vi "Set Event HMI.vi"(8 "error in (no error)":errorcluster caption="entrée d'erreur (pas d'erreur)", 10 "Event HMI":T1, 11 "Sequencer (Default) en entrée":refnum<class "Sequencer (Default).lvclass">) -> (0 "error out":errorcluster caption="sortie d'erreur", 3 "Sequencer (Default) en sortie":refnum<class "Sequencer (Default).lvclass">)   [LabVIEW 2020, in "Library Core.lvlib" / "Sequencer (Default).lvclass"]
uses:
  Sequencer (Default).lvclass
  Software/Standard TB/Function/Type DEF/Commande Gestion Execution Scenario.ctl
  Commun VI/TypeDef/Commande Test/Commande Value Type.ctl
  Commun VI/TypeDef/Commande Test/Commande Type Test.ctl
  Sequencer (Default).lvclass/Sequencer (Default).ctl
  Commun VI/Library Commun.lvlib
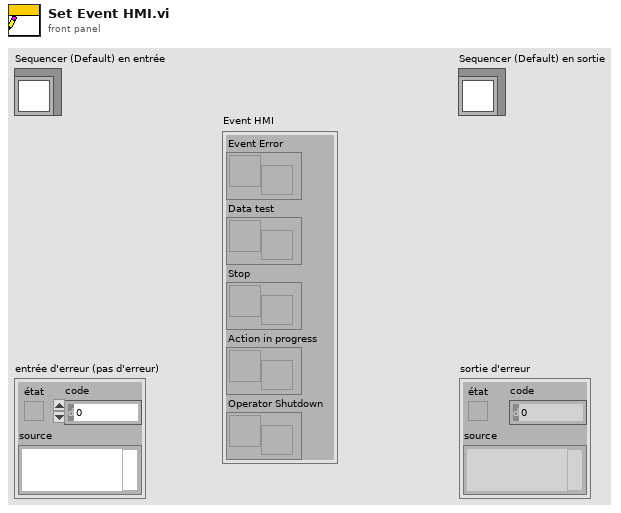
[diagram p1: front panel]
types:
  T1 = cluster{"Event Error":refnum<user-event>, "Data test ":refnum<user-event>, "Stop":refnum<user-event>, "Action in progress":refnum<user-event>, "Operator Shutdown":refnum<user-event>}
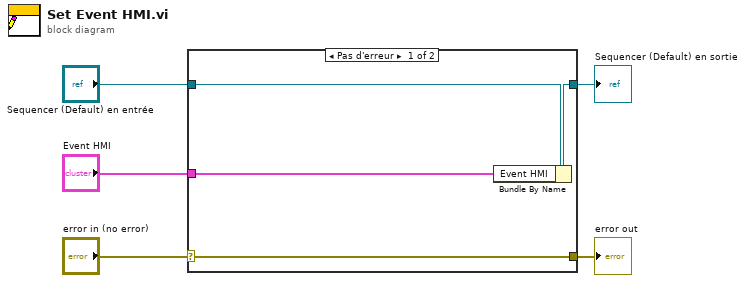
[diagram p0: block diagram]
diagram:
  n1 = case shown="Pas d'erreur" "error in (no error)" {
    selector: "error in (no error)" -> [w9 w10]
    tunnel: [w9 w10] -> w4
    tunnel: [w7 w11] -> w2
    tunnel: "Sequencer (Default) en entrée" -> [w8 w11]
    tunnel: "Event HMI" -> [w6 _]
    frame No Error {
      n2 = Bundle By Name(cluster=w8, "Event HMI"=w6) -> (w7:refnum<class "Sequencer (Default).lvclass">)
    }
    frame Error {
    }
  }
  "error out" <- w4
  "Sequencer (Default) en sortie" <- w2
